vi "Do Core.vi"(8 "error in (no error)":errorcluster, 10 "Actor in":refnum<class "Actor.lvclass">, 11 "Message":refnum<class "Iteration Msg.lvclass">) -> (0 "error out":errorcluster, 2 "Actor out":refnum<class "Actor.lvclass">, 3 "Iterate":bool)   [LabVIEW 2023, in "Example Iterator NR Actor Implicit Iteration.lvlib" / "Iteration Msg.lvclass"]
doc: "(<B>Filename</B>: Actor Framework.lvlib:Reply Msg.lvclass:Do Core.vi)\n\nDefines what an actor does when it receives <B>Reply Message</B>. This method also defines the <B>Reply</B> that is returned to the actor that sent <B>Reply Message</B>.\n\nBy default, this method does nothing, and <B>Reply</B> is the ancestor Message class. A child class must override this method to define behavior and specify a child of the Message class to return in the <B>Reply</B> output."
uses:
  Iteration Msg.lvclass
  <vilib>/ActorFramework/Actor/Actor.lvclass
  Example Actor/Example Actor.lvclass
  C:/Program Files/National Instruments/LabVIEW 2023/vi.lib/ActorFramework/Actor/Actor.lvclass
  Iteration Msg.lvclass/Iteration Msg.ctl
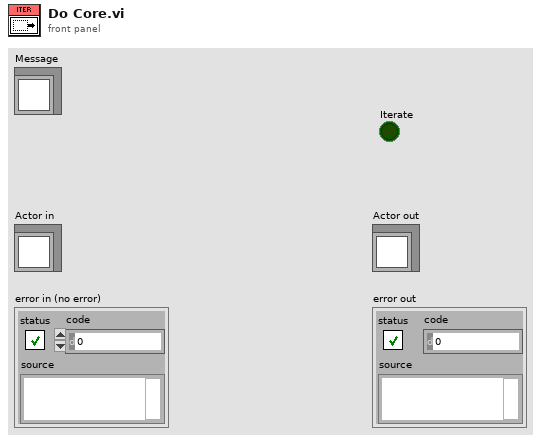
[diagram p1: front panel]
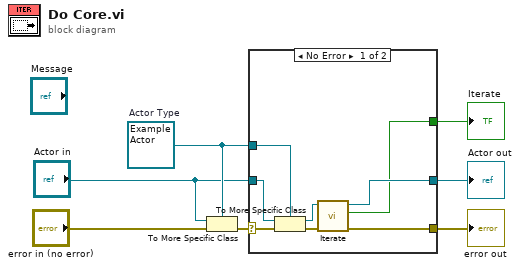
[diagram p0: block diagram]
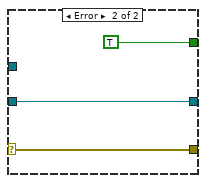
[diagram p2: hidden frame]
diagram:
  w6 = refnum<class "Example Actor.lvclass"> refnum  # Actor Type
  n1 = To More Specific Class(target class=w6, reference="Actor in", error in="error in (no error)") -> (error out=w7:errorcluster)  [unwired: 1 out]
  n2 = case shown="No Error" w7 {
    selector: w7 -> [w15 w18]
    tunnel: [w10 w18] -> w2
    tunnel: [w9 w17] -> w3
    tunnel: "Actor in" -> [w14 w17]
    tunnel: w6 -> [w13 _]
    tunnel: [w8 TRUE ("Continue")] -> w1
    frame No Error {
      n3 = To More Specific Class ("Actor Cast")(target class=w13, reference=w14, error in=w15) -> (specific class reference=w12:refnum<class "Example Actor.lvclass">, error out=w11:errorcluster)
      n4 = call "Iterate.vi"("error in (no error)"=w11, "Example Actor in"=w12) -> ("error out"=w10:errorcluster, "Continue"=w8:bool, "Example Actor out"=w9:refnum<class "Example Actor.lvclass">)  [unwired: 7 in]
    }
    frame Error {
    }
  }
  "error out" <- w2
  "Actor out" <- w3
  "Iterate" <- w1
